vi "generefrekvenssignal0.3.vi"() -> ()   [LabVIEW 2014]
uses:
  <vilib>/MakerHub/LINX/LMH-LINX.lvlib
  <vilib>/MakerHub/LINX/Public/Utilities/Open Serial.vi
  <vilib>/MakerHub/LINX/Public/Peripherals/Analog/Analog Read 1 Chan.vi
panel:
  out "Waveform Graph":dbl[](graph)
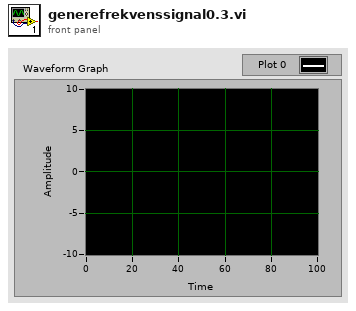
[diagram p1: front panel]
types:
  T1 = typedef "LMH-LINX.lvlib/LINX Ref.ctl" = cluster{"IO":T2, "Interface":T3, "LINX Device Config":T4}
  T2 = typedef "LMH-LINX.lvlib/Platform.ctl" = enum16{"Remote", "Local"}
  T3 = typedef "LMH-LINX.lvlib/Interface.ctl" = enum16{"Serial", "TCP"}
  T4 = typedef "LMH-LINX.lvlib/Device.lvlib/LINX Device Config.ctl" = cluster{"Interface":T3, "COM Port":refnum<visa-resource-name>, "TCP Configuration":T5, "Device Family":u8, "Device ID":u8, "Device Name":string, "TCP Ref":refnum<k5>, "Channels":T6}
  T5 = typedef "LMH-LINX.lvlib/Device.lvlib/TCP Config.ctl" = cluster{"IP Address":string, "Port":u16}
  T6 = typedef "LMH-LINX.lvlib/Channels.ctl" = cluster{"DI":u8[], "DO":u8[], "AI":u8[], "AO":u8[], "PWM":u8[], "QE":u8[], "UART":u8[], "I2C 2":u8[], "SPI":u8[], "CAN":u8[], "Servo":u8[], "AI Ref (V)":dbl, "AI Resolution (Bits)":u8, "AO Ref (V)":dbl, "AO Resolution (Bits)":u8}
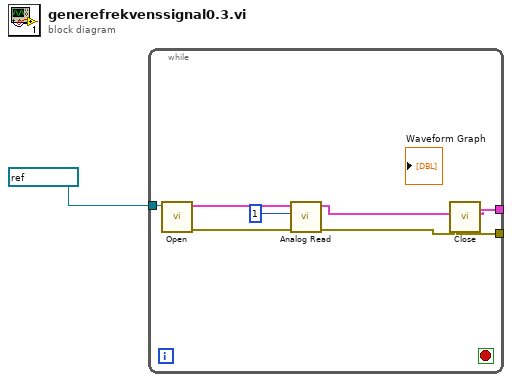
[diagram p0: block diagram]
diagram:
  n1 = while {
    tunnel: [w9] -> w3
    tunnel: refnum<visa-resource-name> "Højtaler" ("Serial Port") -> [w7]
    tunnel: [w5] -> w1
    stop <- _ stop-if-true
    n2 = call-poly <vilib>:"Open.vi"("Serial Port"=w7) -> ("Error Out"=w8:errorcluster, "LINX Resource"=w6:T1)  [unwired: 8 in, 1 out]
    n3 = call-poly <vilib>:"Analog Read.vi"("Error In"=w8, "Analog Channel"=u8 1, "LINX Resource"=w6) -> ("Error Out"=w9:errorcluster, "LINX Resource"=w5:T1)  [unwired: 5 in, 2 out]
  }
  n4 = call <vilib>:"Close.vi"("Error In"=w3, "LINX Resource"=w1) -> ()  [unwired: 9 in, 1 out]
